vi "Move Cursor With Keys.vi"(0 "XYGraph in":refnum<vi>, 1 "index in":i32, 5 "X":dbl[](array[numeric]), 7 "plotIndex":i32, 9 "ScanCode":i16, 11 "Control?":bool) -> (3 "index out":i32, 4 "X":dbl, 6 "Y":dbl, 10 "moved":bool)   [LabVIEW 2020, in "Interactive Graph.xctl"]
uses:
  Interactive Graph.xctl
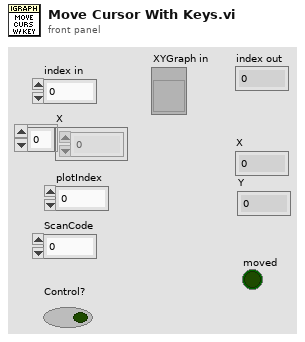
[diagram p1: front panel]
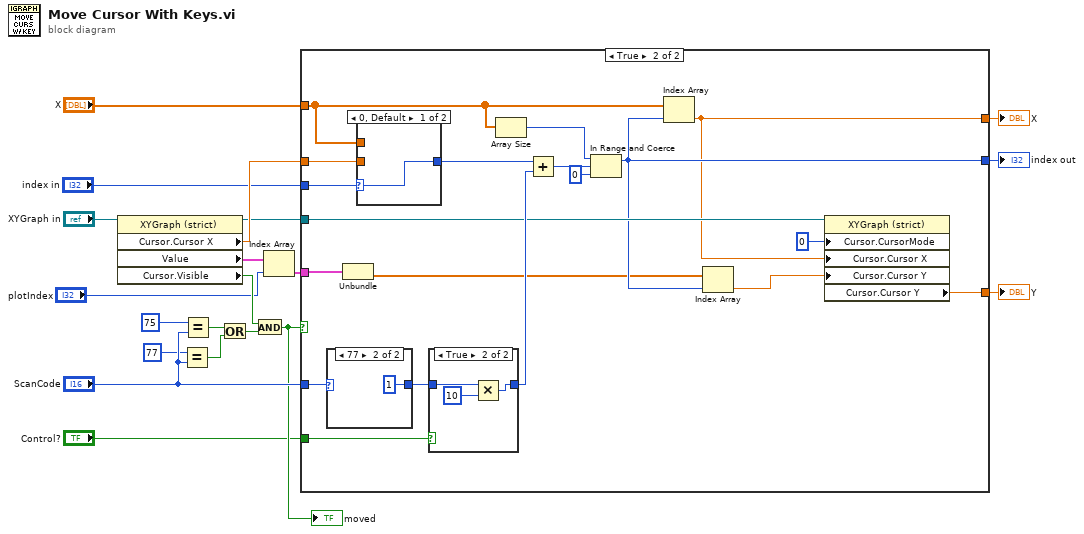
[diagram p0: block diagram]
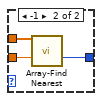
[diagram p3: hidden frame]
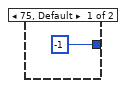
[diagram p5: hidden frame]
diagram:
  n1 = property class="XYGraph (strict)"(reference="XYGraph in") -> (reference out=w8:refnum<vi>, "Cursor.Cursor X"=w10:dbl, "Value"=w3:cluster{dbl[], dbl[]}[], "Cursor.Visible"=w11:bool)  [unwired: 1 in, 1 out]
  n2 = Equal?(x=77, y="ScanCode") -> (x = y?=w14:bool)
  n3 = Equal?(x=75, y="ScanCode") -> (x = y?=w15:bool)
  n4 = Or(x=w15, y=w14) -> (x .or. y?=w13:bool)
  n5 = And(x=w11, y=w13) -> (x .and. y?=w12:bool)
  "moved" <- w12
  n6 = Index Array(array=w3, index="plotIndex") -> (element=w2:cluster{dbl[], dbl[]})
  n7 = case shown="True" w12 {
    tunnel: "X" -> [_ w30]
    tunnel: "ScanCode" -> [_ w39]
    tunnel: w10 -> [_ w40]
    tunnel: "Control?" -> [_ w38]
    tunnel: w8 -> [_ w31]
    tunnel: [_ w23] -> w7
    tunnel: [_ w24] -> w6
    tunnel: "index in" -> [w21 w29]
    tunnel: [w21 w28] -> w4
    tunnel: w2 -> [_ w26]
    frame False {
    }
    frame True {
      n8 = case shown="77" w39 {
        tunnel: [-1 1] -> w37
        frame 75, Default {
        }
        frame 77 {
        }
      }
      n9 = Unbundle(w26) -> (w25:dbl[])  [unwired: 1 out]
      n10 = case shown="0, Default" w29 {
        selector: w29 -> [w41 _]
        tunnel: w40 -> [_ w44]
        tunnel: [w41 w43] -> w36
        tunnel: w30 -> [_ w42]
        frame 0, Default {
        }
        frame -1 {
          n11 = call "Array-Find Nearest.vi"("X"=w42, "U"=w44) -> ("index"=w43:i32)  [unwired: 11 in, 2 out]
        }
      }
      n12 = case shown="True" w38 {
        tunnel: w37 -> [w45 w48]
        tunnel: [w45 w46] -> w35
        frame False {
        }
        frame True {
          n13 = Multiply(x=w48, y=10) -> (x*y=w46:i32)
        }
      }
      n14 = Array Size(array=w30) -> (size(s)=w32:i32)
      n15 = Add(x=w36, y=w35) -> (x+y=w34:i32)
      n16 = In Range and Coerce(upper limit=w32, x=w34, lower limit=0) -> (coerced(x)=w28:i32)  [unwired: 1 out]
      n17 = Index Array(array=w30, index=w28) -> (element=w23:dbl)
      n18 = Index Array(array=w25, index=w28) -> (element=w27:dbl)
      n19 = property class="XYGraph (strict)"(reference=w31, "Cursor.CursorMode"=u32 0 ("Cursor.Cursor Mode"), "Cursor.Cursor X"=w23, "Cursor.Cursor Y"=w27) -> ("Cursor.Cursor Y"=w24:dbl)  [unwired: 1 in, 2 out]
    }
  }
  "X" <- w7
  "Y" <- w6
  "index out" <- w4
